vi "Chart-Multi.vi"() -> ()   [LabVIEW 2020]
panel:
  in  "Delay":u32=100
  out "Chart-Strip":cluster{dbl, dbl}(graph)
  in  "Stop":bool
  # "ms"
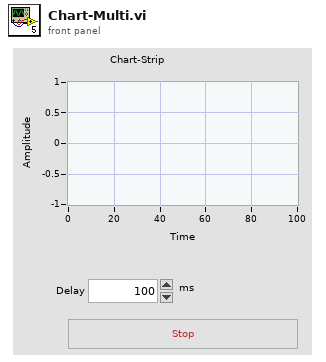
[diagram p1: front panel]
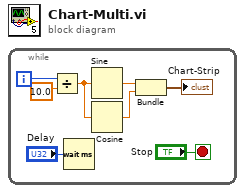
[diagram p0: block diagram]
diagram:
  n1 = while {
    i -> [w7]
    stop <- "Stop" stop-if-true
    n2 = Divide(x=w7, y=10.0 ("x")) -> (x/y=w4:dbl)
    n3 = Wait (ms)(milliseconds to wait="Delay") -> ()  [unwired: 1 out]
    n4 = Sine(x=w4) -> (sin(x)=w3:dbl)
    n5 = Cosine(x=w4) -> (cos(x)=w2:dbl)
    n6 = Bundle(w3, w2) -> (→"Chart-Strip":cluster{dbl, dbl})  [unwired: 1 in]
  }
